vi "Lineup.vi"() -> ()   [LabVIEW 2014]
uses:
  Begin/Global RefNums.vi
  <vilib>/Rock Robotics/WPI/Ultrasonic/WPI_SonarMB1010AnalogRefNum Registry Get.vi
  Begin/Global Variables.vi
  <vilib>/Rock Robotics/WPI/Ultrasonic/WPI_SonarMB1010AnalogGetRange.vi
  <vilib>/addons/control/pid/pid.llb/PID (DBL).vi
  <vilib>/addons/control/pid/NI_PID_pid.lvlib
panel:
  in  "Angle PID gains":T1={"proportional gain (Kc)"=0.1, "integral time (Ti, min)"=0.0, "derivative time (Td, min)"=0.0} {"derivative time (Td, min)" format="%.3f"; "integral time (Ti, min)" format="%.3f"; "proportional gain (Kc)" format="%.3f"}
  in  "Angle output range":cluster{"output high":dbl, "output low":dbl}={"output high"=1.0, "output low"=-1.0} {"output low" format="%.2f"; "output high" format="%.2f"}
  in  "Forward Output Range":cluster{"output high":dbl, "output low":dbl}={"output high"=1.0, "output low"=-1.0} {"output low" format="%.2f"; "output high" format="%.2f"}
  in  "Forward PID gains":T1={"proportional gain (Kc)"=0.05, "integral time (Ti, min)"=0.0, "derivative time (Td, min)"=0.0} {"derivative time (Td, min)" format="%.3f"; "integral time (Ti, min)" format="%.3f"; "proportional gain (Kc)" format="%.3f"}
  in  "Side Range":dbl=0.3
  in  "Side":dbl=20.0 format="%.2f"
  in  "Forward Range":dbl=0.3
  in  "Forward":dbl=15.0 format="%.2f"
  in  "Angle Range":dbl=0.15 format="%#_13g"
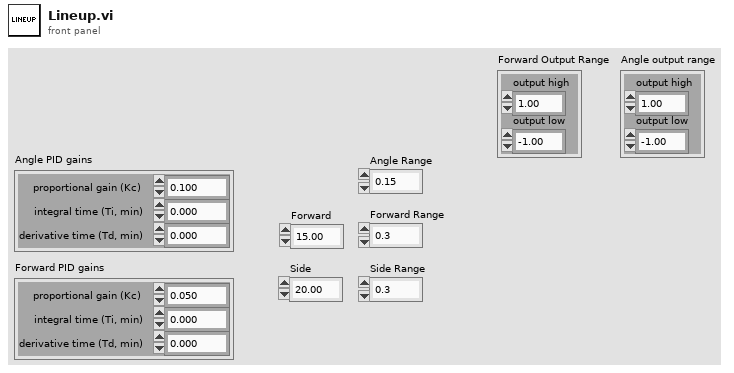
[diagram p1: front panel]
types:
  T1 = cluster{"proportional gain (Kc)":dbl, "integral time (Ti, min)":dbl, "derivative time (Td, min)":dbl}
  T2 = typedef "WPI_SonarMB1010AnalogDeviceRef.ctl" = cluster{"AIDeviceRef":T3, "Scaling factor (V/in)":dbl, "Average Bits":u8}
  T3 = typedef "WPI_AnalogChannelDevRef.ctl" = cluster{"DevStatus":errorcluster, "Controller":T4, "Analog Channel":T5}
  T4 = typedef "FPGA_TypedefAnalogModule.ctl" = enum16{"Controller 1"}
  T5 = typedef "FPGA_AIChannel.ctl" = enum8{"AI 0", "AI 1", "AI 2", "AI 3", "AI MXP 0", "AI MXP 1", "AI MXP 2", "AI MXP 3", "Invalid"}
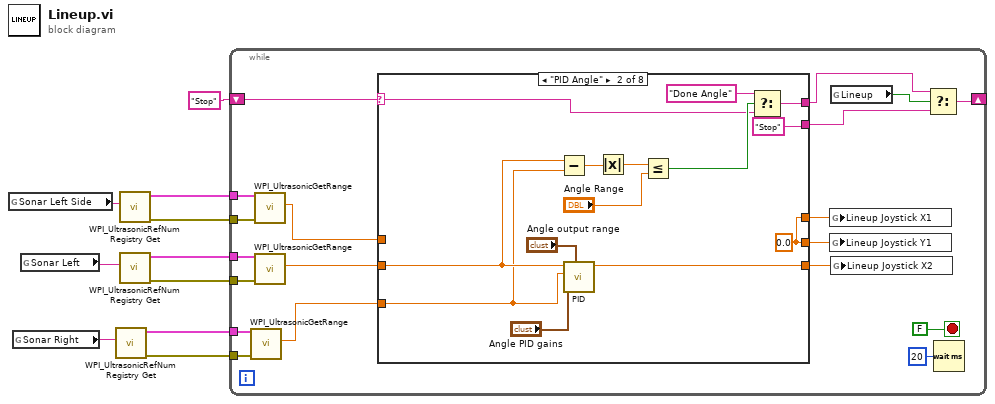
[diagram p0: block diagram]
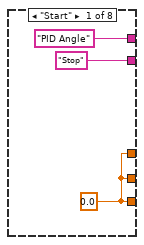
[diagram p2: hidden frame]
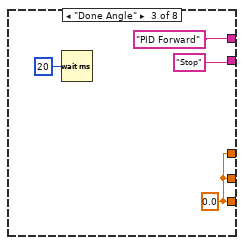
[diagram p3: hidden frame]
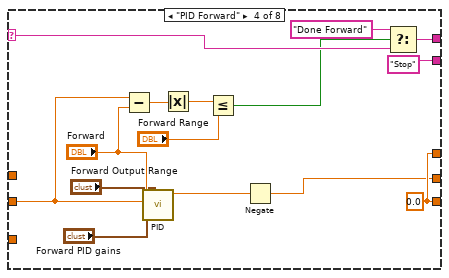
[diagram p4: hidden frame]
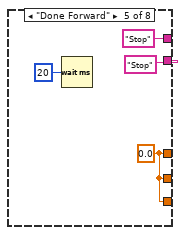
[diagram p5: hidden frame]
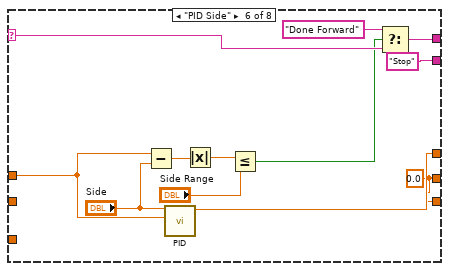
[diagram p6: hidden frame]
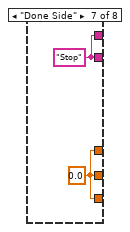
[diagram p7: hidden frame]
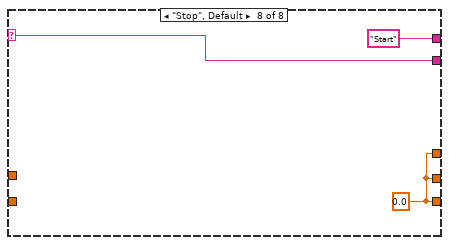
[diagram p8: hidden frame]
diagram:
  n1 = global read "Global RefNums.vi" "Sonar Left Side"() -> (w3:string)
  n2 = global read "Global RefNums.vi" "Sonar Right"() -> (w5:string)
  n3 = global read "Global RefNums.vi" "Sonar Left"() -> (w4:string)
  n4 = call-poly <vilib>:"WPI_UltrasonicRefNum Registry Get.vi"("refnum name"=w5) -> ("error out"=w7:errorcluster, "SonarMB1010AnalogDevRef"=w6:T2)  [unwired: 9 in]
  n5 = call-poly <vilib>:"WPI_UltrasonicRefNum Registry Get.vi"("refnum name"=w3) -> ("error out"=w2:errorcluster, "SonarMB1010AnalogDevRef"=w1:T2)  [unwired: 9 in]
  n6 = call-poly <vilib>:"WPI_UltrasonicRefNum Registry Get.vi"("refnum name"=w4) -> ("error out"=w8:errorcluster, "SonarMB1010AnalogDevRef"=w9:T2)  [unwired: 9 in]
  n7 = while {
    shift-right: [w17] -> _
    shift-left: "Stop" -> [w28]
    tunnel: w9 -> [w24]
    tunnel: w8 -> [w23]
    tunnel: w6 -> [w21]
    tunnel: w7 -> [w22]
    tunnel: w1 -> [w12]
    tunnel: w2 -> [w13]
    stop <- FALSE stop-if-true
    n8 = call-poly <vilib>:"WPI_UltrasonicGetRange.vi"("error in"=w22, "SonarMB1010AnalogDevRef"=w21) -> ("Distance"=w19:dbl)  [unwired: 7 in, 2 out]
    n9 = call-poly <vilib>:"WPI_UltrasonicGetRange.vi"("error in"=w13, "SonarMB1010AnalogDevRef"=w12) -> ("Distance"=w11:dbl)  [unwired: 7 in, 2 out]
    n10 = call-poly <vilib>:"WPI_UltrasonicGetRange.vi"("error in"=w23, "SonarMB1010AnalogDevRef"=w24) -> ("Distance"=w20:dbl)  [unwired: 7 in, 2 out]
    n11 = case shown="\"PID Angle\"" w28 {
      selector: w28 -> [_ w39 _ w60 _ w75 _ w85]
      tunnel: ["PID Angle" ("t") w38 "PID Forward" ("t") w59 "Stop" ("t") w76 w82 "Start" ("t")] -> w16
      tunnel: [w32 w35 w47 w55 w68 w72 w83 w86] -> w27
      tunnel: [w32 w35 w47 w51 w68 w71 w83 w86] -> w26
      tunnel: [w32 w46 w47 w55 w68 w71 w83 w86] -> w25
      tunnel: w20 -> [_ w45 _ w63 _ _ _ _]
      tunnel: w19 -> [_ w44 _ _ _ _ _ _]
      tunnel: ["Stop" ("t") "Stop" ("t") "Stop" ("t") "Stop" ("t") "Stop" ("t") "Stop" ("t") w82 w85] -> w15
      tunnel: w11 -> [_ _ _ _ _ w73 _ _]
      frame "Start" {
        w32 = 0.0 ("Lineup Joystick X2")
      }
      frame "PID Angle" {
        w35 = 0.0 ("Lineup Joystick X2")
        n12 = Subtract(x=w45, y=w44) -> (x-y=w43:dbl)
        n13 = call-poly <vilib>:"PID.vi"("output range"="Angle output range", "PID gains"="Angle PID gains", "process variable"=w44, "setpoint"=w45) -> ("output"=w46:dbl)  [unwired: 6 in, 1 out]
        n14 = Absolute Value(x=w43) -> (abs(x)=w42:dbl)
        n15 = Less Or Equal?(x=w42, y="Angle Range") -> (x <= y?=w40:bool)
        n16 = Select(t="Done Angle", s=w40, f=w39) -> (s? t:f=w38:string)
      }
      frame "Done Angle" {
        w47 = 0.0 ("Lineup Joystick X2")
        n17 = Wait (ms)(milliseconds to wait=u32 20) -> ()  [unwired: 1 out]
      }
      frame "PID Forward" {
        w55 = 0.0 ("Lineup Joystick X2")
        n18 = Subtract(x=w63, y="Forward") -> (x-y=w65:dbl)
        n19 = call-poly <vilib>:"PID.vi"("output range"="Forward Output Range", "PID gains"="Forward PID gains", "process variable"=w63, "setpoint"="Forward") -> ("output"=w52:dbl)  [unwired: 6 in, 1 out]
        n20 = Absolute Value(x=w65) -> (abs(x)=w64:dbl)
        n21 = Less Or Equal?(x=w64, y="Forward Range") -> (x <= y?=w58:bool)
        n22 = Negate(x=w52) -> (-x=w51:dbl)
        n23 = Select(t="Done Forward", s=w58, f=w60) -> (s? t:f=w59:string)
      }
      frame "Done Forward" {
        w68 = 0.0 ("Lineup Joystick X2")
        n24 = Wait (ms)(milliseconds to wait=u32 20) -> ()  [unwired: 1 out]
      }
      frame "PID Side" {
        w71 = 0.0 ("Lineup Joystick X2")
        n25 = Subtract(x=w73, y="Side") -> (x-y=w81:dbl)
        n26 = call-poly <vilib>:"PID.vi"("process variable"=w73, "setpoint"="Side") -> ("output"=w72:dbl)  [unwired: 8 in, 1 out]
        n27 = Absolute Value(x=w81) -> (abs(x)=w80:dbl)
        n28 = Less Or Equal?(x=w80, y="Side Range") -> (x <= y?=w74:bool)
        n29 = Select(t="Done Forward", s=w74, f=w75) -> (s? t:f=w76:string)
      }
      frame "Done Side" {
        w82 = "Stop" ("t")
        w83 = 0.0 ("Lineup Joystick X2")
      }
      frame "Stop", Default {
        w86 = 0.0 ("Lineup Joystick X2")
      }
    }
    n30 = global write "Global Variables.vi" "Lineup Joystick X1"(w27) -> ()
    n31 = global write "Global Variables.vi" "Lineup Joystick Y1"(w26) -> ()
    n32 = global read "Global Variables.vi" "Lineup"() -> (w14:bool)
    n33 = global write "Global Variables.vi" "Lineup Joystick X2"(w25) -> ()
    n34 = Select(t=w16, s=w14, f=w15) -> (s? t:f=w17:string)
    n35 = Wait (ms)(milliseconds to wait=u32 20) -> ()  [unwired: 1 out]
  }
